vi "Main XY Test.vi"() -> ()   [LabVIEW 2017]
uses:
  C:/Program Files (x86)/National Instruments/LabVIEW 2017/examples/Instrument IO/Serial/support/Serial - Settings.ctl
  <vilib>/Instr/_visa.llb/VISA Configure Serial Port (Instr).vi
panel:
  in  "XY_M_MotorOff":bool
  in  "XY_M_MotorOn":bool
  in  "XY_L_X":bool
  in  "XY_L_KonKreise":bool
  in  "XY_M_Center":bool
  in  "XY_L_Kreis_X":bool
  in  "Y rel":i32
  in  "X rel":i32
  in  "XY_M_Relative":bool
  in  "Y":i32 min=0 max=15000
  in  "X":i32 min=0 max=15000
  in  "XY_M_Move":bool
  in  "XY_M_Trigger":bool
  in  "Stopp":bool
  out "Antwort":string
  in  "VISA-Ressourcenname":refnum<visa-resource-name>="COM13"
  in  "Einstellungen des seriellen Ports":T1={"Baudrate"=19200, "Datenbits"=8, "Parität"=enum."None", "Stoppbits"=10, "Ablaufsteuerung"=0} {"Ablaufsteuerung" items=["Keine"=0, "XON/XOFF"=1, "RTS/CTS"=2, "DTR/DSR"=4]; "Stoppbits" items=["1,0"=10, "1,5"=15, "2,0"=20]; "Datenbits" min=5 max=8 step=1; "Baudrate" items=["75"=75, "110"=110, "134"=134, "150"=150, "300"=300, "600"=600, "1200"=1200, "1800"=1800, "2400"=2400, "4800"=4800, "7200"=7200, "9600"=9600, "14400"=14400, "19200"=19200, "28800"=28800, "38400"=38400, "56000"=56000, "57600"=57600, "115200"=115200, "128000"=128000, "230400"=230400]}
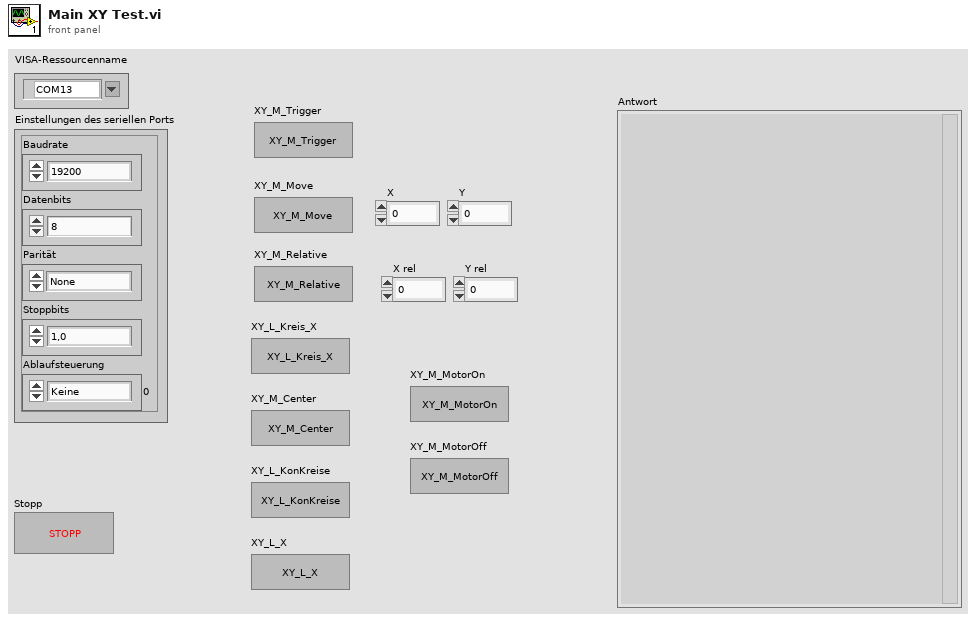
[diagram p1: front panel]
types:
  T1 = typedef "Serial - Settings.ctl" = cluster{"Baudrate":u32, "Datenbits":u16, "Parität":enum16{"None", "Odd", "Even", "Mark", "Space"}, "Stoppbits":u16, "Ablaufsteuerung":u16}
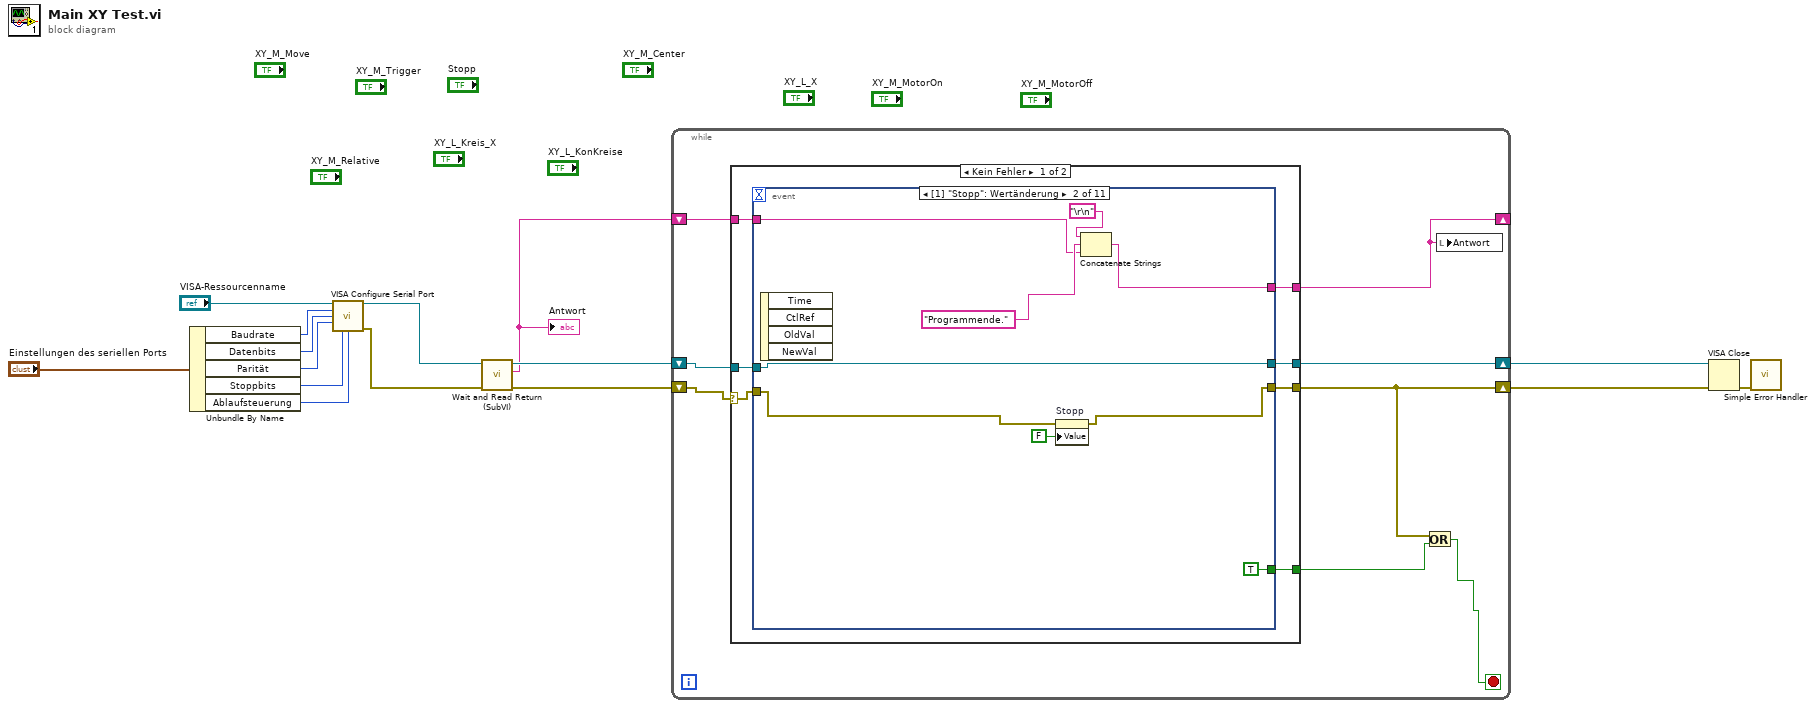
[diagram p0: block diagram]
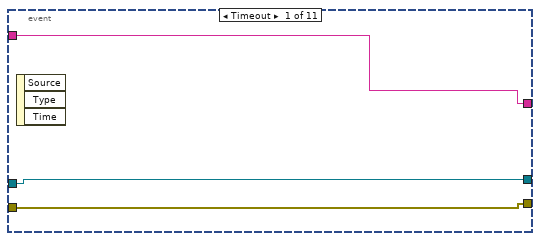
[diagram p2: hidden frame]
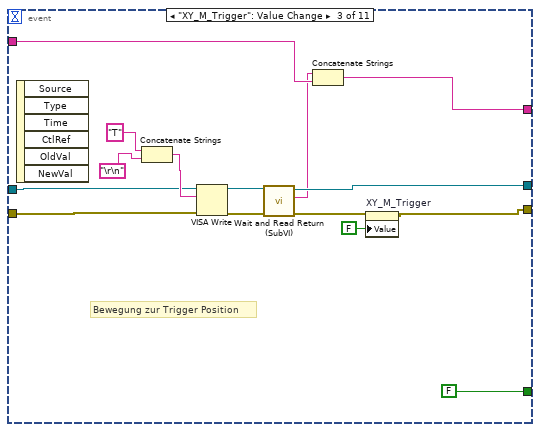
[diagram p3: hidden frame]
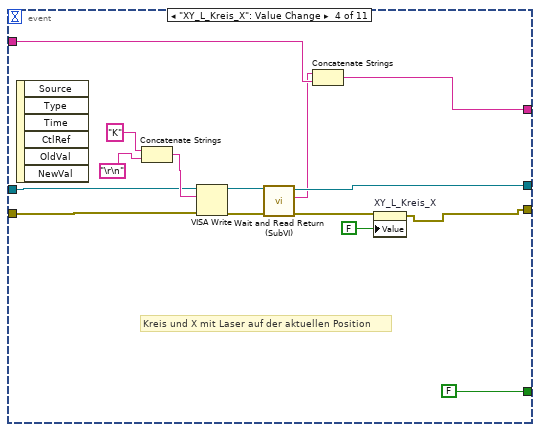
[diagram p4: hidden frame]
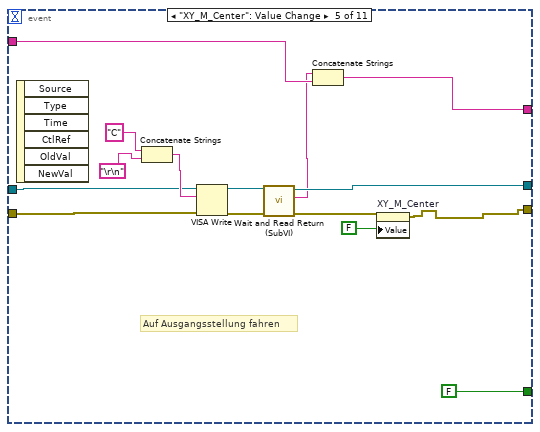
[diagram p5: hidden frame]
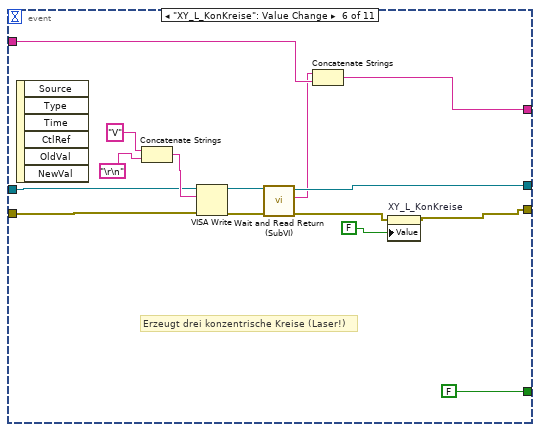
[diagram p6: hidden frame]
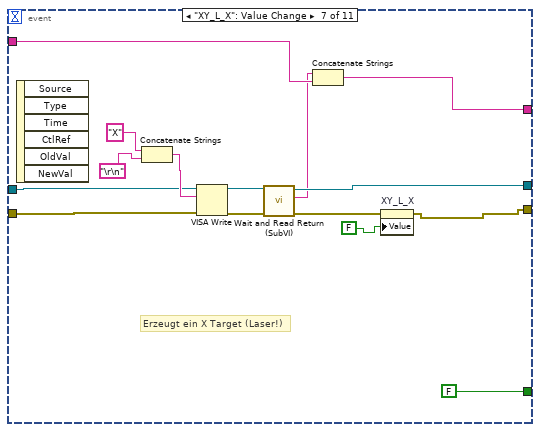
[diagram p7: hidden frame]
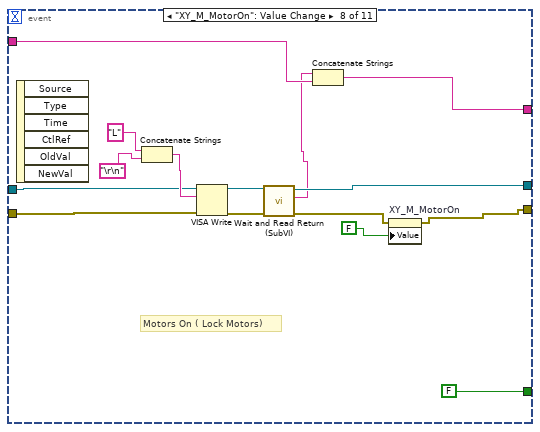
[diagram p8: hidden frame]
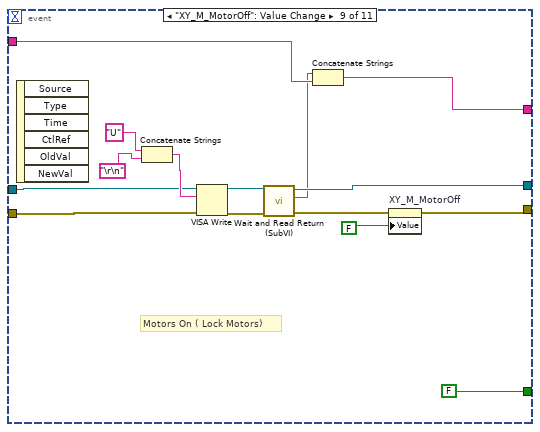
[diagram p9: hidden frame]
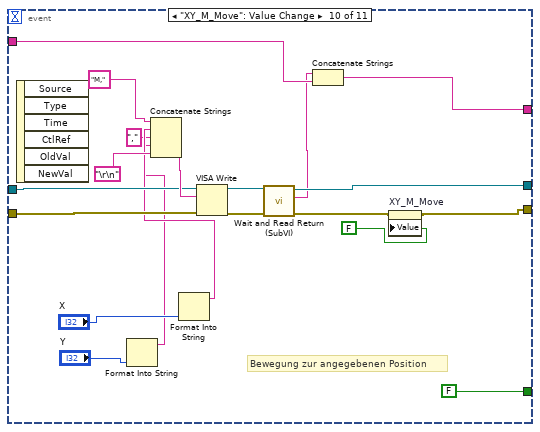
[diagram p10: hidden frame]
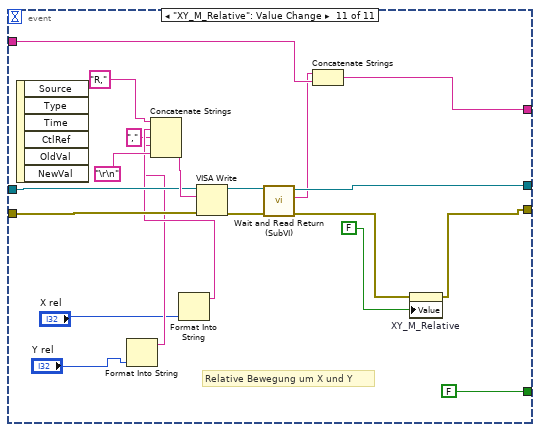
[diagram p11: hidden frame]
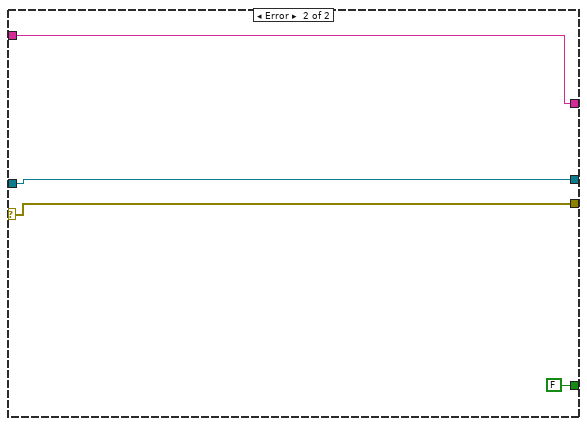
[diagram p12: hidden frame]
diagram:
  n1 = Unbundle By Name("Einstellungen des seriellen Ports") -> ("Baudrate"=w10:u32, "Datenbits"=w11:u16, "Parität"=w12:enum16{"None", "Odd", "Even", "Mark", "Space"}, "Stoppbits"=w13:u16, "Ablaufsteuerung"=w8:u16)
  n2 = call-poly "VISA Configure Serial Port"("VISA resource name"="VISA-Ressourcenname", "baud rate (9600)"=w10, "data bits (8)"=w11, "parity (0:none)"=w12, "stop bits (10: 1 bit)"=w13, "flow control (0:none)"=w8) -> ("VISA resource name out"=w7:refnum<visa-resource-name>, "error out"=w6:errorcluster)  [unwired: 4 in, 4 out]
  n3 = call "Wait and Read Return (SubVI).vi"("Fehler (Eingang, kein Fehler)"=w6, "VISA-Referenz (Eingang)"=w7) -> ("Fehler (Ausgang)"=w4:errorcluster, "Antwort"=w1:string, "VISA-Referenz (Ausgang)"=w5:refnum<visa-resource-name>)  [unwired: 7 in]
  "Antwort" <- w1
  n4 = while {
    shift-right: [w22] -> w3
    shift-left: w5 -> [w23]
    shift-right: [w19] -> w2
    shift-left: w4 -> [w16]
    shift-right: [w20] -> _
    shift-left: w1 -> [w21]
    stop <- w17 stop-if-true
    n5 = case shown="Kein Fehler" w16 {
      selector: w16 -> [w24 w191]
      tunnel: w23 -> [w30 w190]
      tunnel: [w29 w190] -> w22
      tunnel: w21 -> [w28 w189]
      tunnel: [w27 w189] -> w20
      tunnel: [w26 w191] -> w19
      tunnel: [w25 FALSE] -> w18
      frame No Error {
        n6 = event shown="[1] \"Stopp\": Wertänderung" {
          selector: _ -> [_ _ _ _ _ _ _ _ _ _ _]
          dyn-events: _ -> [_ _ _ _ _ _ _ _ _ _ _]
          timeout: _ -> [_ _ _ _ _ _ _ _ _ _ _]
          tunnel: w30 -> [w33 w42 w52 w67 w82 w97 w112 w127 w142 w163 w183]
          tunnel: w24 -> [w32 w39 w51 w66 w81 w96 w111 w126 w141 w162 w182]
          tunnel: [w33 w42 w50 w65 w80 w95 w110 w125 w140 w161 w181] -> w29
          tunnel: [w32 w38 w45 w60 w75 w90 w105 w120 w135 w152 w172] -> w26
          tunnel: [w31 w40 w48 w63 w78 w93 w108 w123 w138 w159 w179] -> w27
          tunnel: [_ TRUE FALSE FALSE FALSE FALSE FALSE FALSE FALSE FALSE FALSE] -> w25
          tunnel: w28 -> [w31 w35 w44 w59 w74 w89 w104 w119 w134 w149 w169]
          event Timeout {
            n7 = event-data() -> ()  [unwired: 1 in, 3 out]
          }
          event "Stopp": Value Change {
            n8 = event-data() -> ()  [unwired: 1 in, 4 out]
            n9 = property on="Stopp" class="Bool. (strikt)"(error in=w39, "Value"=FALSE ("Stopp")) -> (error out=w38:errorcluster)  [unwired: 1 in, 1 out]
            n10 = Concatenate Strings("\r\n", "Programmende." ("String"), w35) -> (w40:string)
          }
          event "XY_M_Trigger": Value Change {
            # "Bewegung zur Trigger Position"
            n11 = event-data() -> ()  [unwired: 1 in, 6 out]
            n12 = Concatenate Strings("T" ("Schreibpuffer"), "\r\n") -> (w55:string)
            n13 = VISA Write(VISA resource name=w52, write buffer=w55, error in (no error)=w51) -> (VISA resource name out=w54:refnum<visa-resource-name>, error out=w53:errorcluster)  [unwired: 1 out]
            n14 = call "Wait and Read Return (SubVI).vi"("Fehler (Eingang, kein Fehler)"=w53, "VISA-Referenz (Eingang)"=w54) -> ("Fehler (Ausgang)"=w46:errorcluster, "Antwort"=w43:string, "VISA-Referenz (Ausgang)"=w50:refnum<visa-resource-name>)  [unwired: 7 in]
            n15 = Concatenate Strings(w43, w44) -> (w48:string)
            n16 = property on="XY_M_Trigger" class="Bool. (strikt)"(error in=w46, "Value"=FALSE ("XY_M_Trigger")) -> (error out=w45:errorcluster)  [unwired: 1 in, 1 out]
          }
          event "XY_L_Kreis_X": Value Change {
            # "Kreis und X mit Laser auf der aktuellen Position"
            n17 = event-data() -> ()  [unwired: 1 in, 6 out]
            n18 = Concatenate Strings("K" ("Schreibpuffer"), "\r\n") -> (w70:string)
            n19 = VISA Write(VISA resource name=w67, write buffer=w70, error in (no error)=w66) -> (VISA resource name out=w69:refnum<visa-resource-name>, error out=w68:errorcluster)  [unwired: 1 out]
            n20 = call "Wait and Read Return (SubVI).vi"("Fehler (Eingang, kein Fehler)"=w68, "VISA-Referenz (Eingang)"=w69) -> ("Fehler (Ausgang)"=w61:errorcluster, "Antwort"=w58:string, "VISA-Referenz (Ausgang)"=w65:refnum<visa-resource-name>)  [unwired: 7 in]
            n21 = Concatenate Strings(w58, w59) -> (w63:string)
            n22 = property on="XY_L_Kreis_X" class="Bool. (strikt)"(error in=w61, "Value"=FALSE ("XY_M_Trigger")) -> (error out=w60:errorcluster)  [unwired: 1 in, 1 out]
          }
          event "XY_M_Center": Value Change {
            # "Auf Ausgangsstellung fahren"
            n23 = event-data() -> ()  [unwired: 1 in, 6 out]
            n24 = Concatenate Strings("C" ("Schreibpuffer"), "\r\n") -> (w85:string)
            n25 = VISA Write(VISA resource name=w82, write buffer=w85, error in (no error)=w81) -> (VISA resource name out=w84:refnum<visa-resource-name>, error out=w83:errorcluster)  [unwired: 1 out]
            n26 = call "Wait and Read Return (SubVI).vi"("Fehler (Eingang, kein Fehler)"=w83, "VISA-Referenz (Eingang)"=w84) -> ("Fehler (Ausgang)"=w76:errorcluster, "Antwort"=w73:string, "VISA-Referenz (Ausgang)"=w80:refnum<visa-resource-name>)  [unwired: 7 in]
            n27 = Concatenate Strings(w73, w74) -> (w78:string)
            n28 = property on="XY_M_Center" class="Bool. (strikt)"(error in=w76, "Value"=FALSE ("XY_M_Trigger")) -> (error out=w75:errorcluster)  [unwired: 1 in, 1 out]
          }
          event "XY_L_KonKreise": Value Change {
            # "Erzeugt drei konzentrische Kreise (Laser!)"
            n29 = event-data() -> ()  [unwired: 1 in, 6 out]
            n30 = Concatenate Strings("V" ("Schreibpuffer"), "\r\n") -> (w100:string)
            n31 = VISA Write(VISA resource name=w97, write buffer=w100, error in (no error)=w96) -> (VISA resource name out=w99:refnum<visa-resource-name>, error out=w98:errorcluster)  [unwired: 1 out]
            n32 = call "Wait and Read Return (SubVI).vi"("Fehler (Eingang, kein Fehler)"=w98, "VISA-Referenz (Eingang)"=w99) -> ("Fehler (Ausgang)"=w91:errorcluster, "Antwort"=w88:string, "VISA-Referenz (Ausgang)"=w95:refnum<visa-resource-name>)  [unwired: 7 in]
            n33 = Concatenate Strings(w88, w89) -> (w93:string)
            n34 = property on="XY_L_KonKreise" class="Bool. (strikt)"(error in=w91, "Value"=FALSE ("XY_M_Trigger")) -> (error out=w90:errorcluster)  [unwired: 1 in, 1 out]
          }
          event "XY_L_X": Value Change {
            # "Erzeugt ein X Target (Laser!)"
            n35 = event-data() -> ()  [unwired: 1 in, 6 out]
            n36 = Concatenate Strings("X" ("Schreibpuffer"), "\r\n") -> (w115:string)
            n37 = VISA Write(VISA resource name=w112, write buffer=w115, error in (no error)=w111) -> (VISA resource name out=w114:refnum<visa-resource-name>, error out=w113:errorcluster)  [unwired: 1 out]
            n38 = call "Wait and Read Return (SubVI).vi"("Fehler (Eingang, kein Fehler)"=w113, "VISA-Referenz (Eingang)"=w114) -> ("Fehler (Ausgang)"=w106:errorcluster, "Antwort"=w103:string, "VISA-Referenz (Ausgang)"=w110:refnum<visa-resource-name>)  [unwired: 7 in]
            n39 = Concatenate Strings(w103, w104) -> (w108:string)
            n40 = property on="XY_L_X" class="Bool. (strikt)"(error in=w106, "Value"=FALSE ("XY_M_Trigger")) -> (error out=w105:errorcluster)  [unwired: 1 in, 1 out]
          }
          event "XY_M_MotorOn": Value Change {
            # "Motors On ( Lock Motors)"
            n41 = event-data() -> ()  [unwired: 1 in, 6 out]
            n42 = Concatenate Strings("L" ("Schreibpuffer"), "\r\n") -> (w130:string)
            n43 = VISA Write(VISA resource name=w127, write buffer=w130, error in (no error)=w126) -> (VISA resource name out=w129:refnum<visa-resource-name>, error out=w128:errorcluster)  [unwired: 1 out]
            n44 = call "Wait and Read Return (SubVI).vi"("Fehler (Eingang, kein Fehler)"=w128, "VISA-Referenz (Eingang)"=w129) -> ("Fehler (Ausgang)"=w121:errorcluster, "Antwort"=w118:string, "VISA-Referenz (Ausgang)"=w125:refnum<visa-resource-name>)  [unwired: 7 in]
            n45 = Concatenate Strings(w118, w119) -> (w123:string)
            n46 = property on="XY_M_MotorOn" class="Bool. (strikt)"(error in=w121, "Value"=FALSE ("XY_M_Trigger")) -> (error out=w120:errorcluster)  [unwired: 1 in, 1 out]
          }
          event "XY_M_MotorOff": Value Change {
            # "Motors On ( Lock Motors)"
            n47 = event-data() -> ()  [unwired: 1 in, 6 out]
            n48 = Concatenate Strings("U" ("Schreibpuffer"), "\r\n") -> (w145:string)
            n49 = VISA Write(VISA resource name=w142, write buffer=w145, error in (no error)=w141) -> (VISA resource name out=w144:refnum<visa-resource-name>, error out=w143:errorcluster)  [unwired: 1 out]
            n50 = call "Wait and Read Return (SubVI).vi"("Fehler (Eingang, kein Fehler)"=w143, "VISA-Referenz (Eingang)"=w144) -> ("Fehler (Ausgang)"=w136:errorcluster, "Antwort"=w133:string, "VISA-Referenz (Ausgang)"=w140:refnum<visa-resource-name>)  [unwired: 7 in]
            n51 = Concatenate Strings(w133, w134) -> (w138:string)
            n52 = property on="XY_M_MotorOff" class="Bool. (strikt)"(error in=w136, "Value"=FALSE ("XY_M_Trigger")) -> (error out=w135:errorcluster)  [unwired: 1 in, 1 out]
          }
          event "XY_M_Move": Value Change {
            # "Bewegung zur angegebenen Position"
            n53 = event-data() -> ()  [unwired: 1 in, 6 out]
            n54 = Format Into String("Y") -> (resulting string=w154:string)  [unwired: 3 in, 1 out]
            n55 = Format Into String("X") -> (resulting string=w155:string)  [unwired: 3 in, 1 out]
            n56 = Concatenate Strings("M," ("Schreibpuffer"), w155, "," ("String"), w154, "\r\n") -> (w166:string)
            n57 = VISA Write(VISA resource name=w163, write buffer=w166, error in (no error)=w162) -> (VISA resource name out=w165:refnum<visa-resource-name>, error out=w164:errorcluster)  [unwired: 1 out]
            n58 = call "Wait and Read Return (SubVI).vi"("Fehler (Eingang, kein Fehler)"=w164, "VISA-Referenz (Eingang)"=w165) -> ("Fehler (Ausgang)"=w151:errorcluster, "Antwort"=w148:string, "VISA-Referenz (Ausgang)"=w161:refnum<visa-resource-name>)  [unwired: 7 in]
            n59 = Concatenate Strings(w148, w149) -> (w159:string)
            n60 = property on="XY_M_Move" class="Bool. (strikt)"(error in=w151, "Value"=FALSE ("XY_M_Trigger")) -> (error out=w152:errorcluster)  [unwired: 1 in, 1 out]
          }
          event "XY_M_Relative": Value Change {
            # "Relative Bewegung um X und Y"
            n61 = event-data() -> ()  [unwired: 1 in, 6 out]
            n62 = Format Into String("Y rel") -> (resulting string=w176:string)  [unwired: 3 in, 1 out]
            n63 = Format Into String("X rel") -> (resulting string=w177:string)  [unwired: 3 in, 1 out]
            n64 = Concatenate Strings("R," ("Schreibpuffer"), w177, "," ("String"), w176, "\r\n") -> (w186:string)
            n65 = VISA Write(VISA resource name=w183, write buffer=w186, error in (no error)=w182) -> (VISA resource name out=w185:refnum<visa-resource-name>, error out=w184:errorcluster)  [unwired: 1 out]
            n66 = call "Wait and Read Return (SubVI).vi"("Fehler (Eingang, kein Fehler)"=w184, "VISA-Referenz (Eingang)"=w185) -> ("Fehler (Ausgang)"=w173:errorcluster, "Antwort"=w168:string, "VISA-Referenz (Ausgang)"=w181:refnum<visa-resource-name>)  [unwired: 7 in]
            n67 = Concatenate Strings(w168, w169) -> (w179:string)
            n68 = property on="XY_M_Relative" class="Bool. (strikt)"(error in=w173, "Value"=FALSE ("XY_M_Trigger")) -> (error out=w172:errorcluster)  [unwired: 1 in, 1 out]
          }
        }
      }
      frame Error {
      }
    }
    n69 = Or(x=w19, y=w18) -> (x .or. y?=w17:bool)
    n70 = local write "Antwort"(w20) -> ()
  }
  n71 = VISA Close(VISA resource name=w3, error in (no error)=w2) -> (error out=w15:errorcluster)
  n72 = call <vilib>:"Simple Error Handler.vi"("error in (no error)"=w15) -> ()  [unwired: 4 in, 5 out]
